vi "GFITS_SelectHdrFile.vi"(7 "auxhdr":path=path "", 10 "line in":string, 11 "Database RefNum":T1) -> (1 "path out":path, 2 "line out":string)   [LabVIEW 2016]
uses:
  DBSHAND/private/vis/DatabaseHand_RefNum.ctl
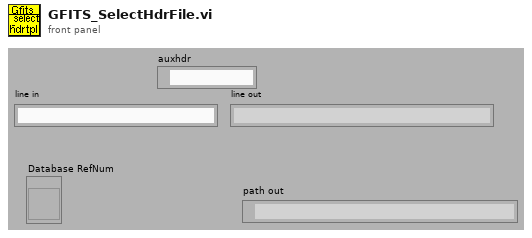
[diagram p1: front panel]
types:
  T1 = typedef "DatabaseHand_RefNum.ctl" = refnum<vi>
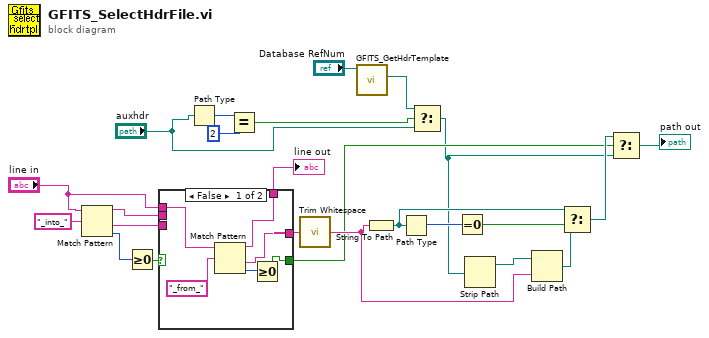
[diagram p0: block diagram]
diagram:
  n1 = Match Pattern(string="line in", regular expression="_into_") -> (before substring=w7:string, after substring=w12:string, offset past match=w22:i32)  [unwired: 2 out]
  n2 = Greater Or Equal To 0?(x=w22) -> (x >= 0?=w13:bool)
  n3 = case shown="False" w13 {
    selector: w13 -> [_ w32]
    tunnel: w12 -> [_ w33]
    tunnel: [w26 w33] -> w11
    tunnel: [w27 w32] -> w10
    tunnel: "line in" -> [w29 _]
    tunnel: [w25 w31] -> w8
    tunnel: w7 -> [_ w31]
    frame False {
      n4 = Match Pattern(string=w29, regular expression="_from_") -> (before substring=w25:string, after substring=w26:string, offset past match=w28:i32)  [unwired: 2 out]
      n5 = Greater Or Equal To 0?(x=w28) -> (x >= 0?=w27:bool)
    }
    frame True {
    }
  }
  "line out" <- w8
  n6 = Path Type(1:"auxhdr") -> (0:w6:i16)
  n7 = Equal?(x=w6, y=i16 2) -> (x = y?=w2:bool)
  n8 = call <vilib>:"Trim Whitespace.vi"("string"=w11) -> ("trimmed string"=w16:string)  [unwired: 1 in]
  n9 = call "GFITS_GetHdrTemplate.vi"("Database RefNum"="Database RefNum") -> ("path"=w4:path)  [unwired: 10 out]
  n10 = String To Path(string=w16) -> (path=w14:path)
  n11 = Path Type(1:w14) -> (0:w21:i16)
  n12 = Select(t=w4, s=w2, f="auxhdr") -> (s? t:f=w3:path)
  n13 = Equal To 0?(x=w21) -> (x = 0?=w20:bool)
  n14 = Strip Path(path=w3) -> (stripped path=w19:path)  [unwired: 1 out]
  n15 = Build Path(base path=w19, name or relative path=w16) -> (appended path=w18:path)
  n16 = Select(t=w14, s=w20, f=w18) -> (s? t:f=w15:path)
  n17 = Select(t=w15, s=w10, f=w3) -> (s? t:f=→"path out":path)
